vi "Flush Control Value.vi"(4 "error in (no error)":errorcluster, 5 "Tab Control Ref In":T2, 6 "Tree Control In":refnum<vi>, 7 "Session In":T1) -> (0 "error out":errorcluster, 2 "Tree Control Out":refnum<vi>, 3 "Session Out":T1)   [LabVIEW 2012]
doc: "The Flush Control Value subVI reads the value of the control, and then sets the value of the attribute in the IMAQdx driver."
uses:
  <vilib>/userDefined/High Color/IMAQdx.ctl
  <vilib>/vision/driver/IMAQdx.llb/IMAQdx Attribute Type.ctl
  <vilib>/vision/driver/NI_Vision_Acquisition_Software.lvlib
  <resource>/objmgr/imaqdx.rc
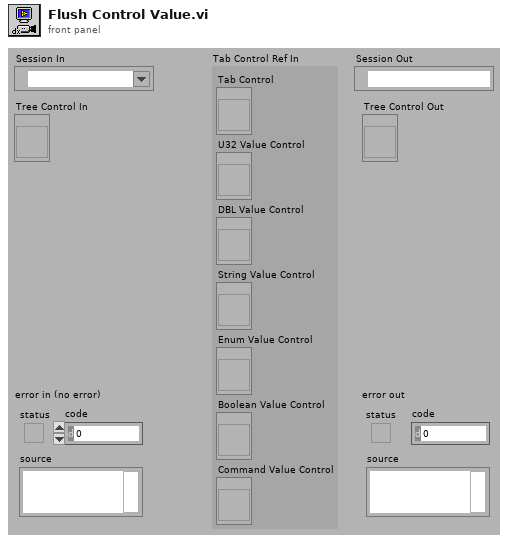
[diagram p1: front panel]
types:
  T1 = typedef "IMAQdx.ctl" = refnum<k21>
  T2 = cluster{"Tab Control":refnum<vi>, "U32 Value Control":refnum<vi>, "DBL Value Control":refnum<vi>, "String Value Control":refnum<vi>, "Enum Value Control":refnum<vi>, "Boolean Value Control":refnum<vi>, "Command Value Control":refnum<vi>}
  T3 = typedef "NI_Vision_Acquisition_Software.lvlib/IMAQdx Attribute Type.ctl" = enum32{"U32", "I64", "DBL", "String", "Enum", "Bool", "Command"}
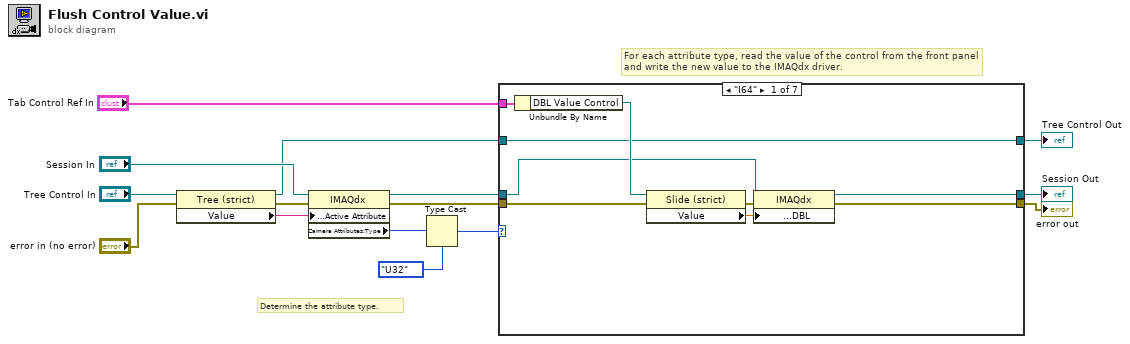
[diagram p0: block diagram]
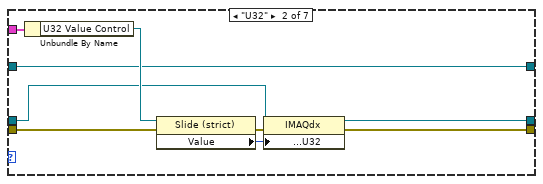
[diagram p2: hidden frame]
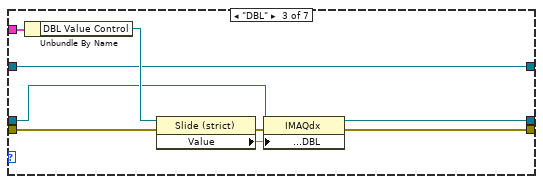
[diagram p3: hidden frame]
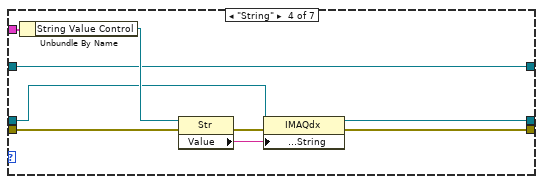
[diagram p4: hidden frame]
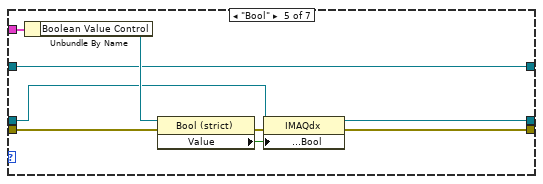
[diagram p5: hidden frame]
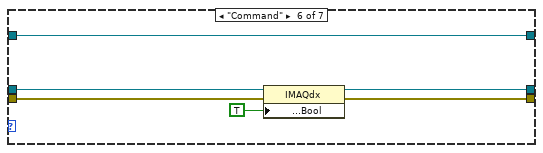
[diagram p6: hidden frame]
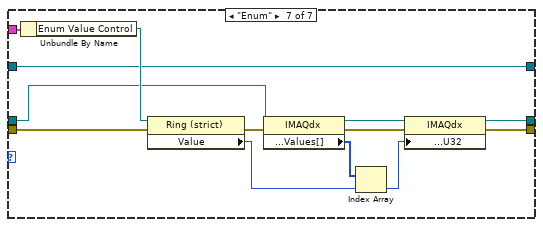
[diagram p7: hidden frame]
diagram:
  # "For each attribute type, read the value of the control from the front panel\nand write the new value to the IMAQdx driver."
  # "Determine the attribute type."
  n1 = property class="Tree (strict)"(reference="Tree Control In", error in="error in (no error)") -> (reference out=w4:refnum<vi>, error out=w13:errorcluster, "Value"=w11:string)
  n2 = property class="IMAQdx"(reference="Session In", error in=w13, "Camera Attributes:Active Attribute"=w11) -> (reference out=w6:T1, error out=w7:errorcluster, "Camera Attributes:Type"=w10:u32)
  n3 = Type Cast(type=IMAQdx_Attribute_Type."U32" ("Attribute Type"), x=w10) -> (*(type *) &x=w8:T3)
  n4 = case shown="\"I64\"" w8 {
    tunnel: w7 -> [w22 w31 w40 w49 w58 w62 w77]
    tunnel: w6 -> [w20 w29 w38 w47 w56 w66 w75]
    tunnel: "Tab Control Ref In" -> [w24 w33 w42 w51 w60 _ w79]
    tunnel: [w18 w27 w36 w45 w54 w65 w73] -> w2
    tunnel: [w17 w26 w35 w44 w53 w64 w72] -> w1
    tunnel: [w16 w25 w34 w43 w52 w63 w74] -> w3
    tunnel: w4 -> [w16 w25 w34 w43 w52 w63 w74]
    frame "I64" {
      n5 = Unbundle By Name(w24) -> ("DBL Value Control"=w23:refnum<vi>)
      n6 = property class="Slide (strict)"(reference=w23, error in=w22) -> (error out=w21:errorcluster, "Value"=w19:dbl)  [unwired: 1 out]
      n7 = property class="IMAQdx"(reference=w20, error in=w21, "Camera Attributes:Value:DBL"=w19) -> (reference out=w18:T1, error out=w17:errorcluster)
    }
    frame "U32" {
      n8 = Unbundle By Name(w33) -> ("U32 Value Control"=w32:refnum<vi>)
      n9 = property class="Slide (strict)"(reference=w32, error in=w31) -> (error out=w30:errorcluster, "Value"=w28:u32)  [unwired: 1 out]
      n10 = property class="IMAQdx"(reference=w29, error in=w30, "Camera Attributes:Value:U32"=w28) -> (reference out=w27:T1, error out=w26:errorcluster)
    }
    frame "DBL" {
      n11 = Unbundle By Name(w42) -> ("DBL Value Control"=w41:refnum<vi>)
      n12 = property class="Slide (strict)"(reference=w41, error in=w40) -> (error out=w39:errorcluster, "Value"=w37:dbl)  [unwired: 1 out]
      n13 = property class="IMAQdx"(reference=w38, error in=w39, "Camera Attributes:Value:DBL"=w37) -> (reference out=w36:T1, error out=w35:errorcluster)
    }
    frame "String" {
      n14 = Unbundle By Name(w51) -> ("String Value Control"=w50:refnum<vi>)
      n15 = property class="Str"(reference=w50, error in=w49) -> (error out=w48:errorcluster, "Value"=w46:string)  [unwired: 1 out]
      n16 = property class="IMAQdx"(reference=w47, error in=w48, "Camera Attributes:Value:String"=w46) -> (reference out=w45:T1, error out=w44:errorcluster)
    }
    frame "Bool" {
      n17 = Unbundle By Name(w60) -> ("Boolean Value Control"=w59:refnum<vi>)
      n18 = property class="Bool (strict)"(reference=w59, error in=w58) -> (error out=w57:errorcluster, "Value"=w55:bool)  [unwired: 1 out]
      n19 = property class="IMAQdx"(reference=w56, error in=w57, "Camera Attributes:Value:Bool"=w55) -> (reference out=w54:T1, error out=w53:errorcluster)
    }
    frame "Command" {
      n20 = property class="IMAQdx"(reference=w66, error in=w62, "Camera Attributes:Value:Bool"=TRUE ("ValueBool")) -> (reference out=w65:T1, error out=w64:errorcluster)
    }
    frame "Enum" {
      n21 = Unbundle By Name(w79) -> ("Enum Value Control"=w78:refnum<vi>)
      n22 = property class="Ring (strict)"(reference=w78, error in=w77) -> (error out=w76:errorcluster, "Value"=w67:u32)  [unwired: 1 out]
      n23 = property class="IMAQdx"(reference=w75, error in=w76) -> (reference out=w71:T1, error out=w70:errorcluster, "Camera Attributes:Enum:Values[]"=w69:u32[])
      n24 = Index Array(array=w69, index=w67) -> (element=w68:u32)
      n25 = property class="IMAQdx"(reference=w71, error in=w70, "Camera Attributes:Value:U32"=w68) -> (reference out=w73:T1, error out=w72:errorcluster)
    }
  }
  "Tree Control Out" <- w3
  "Session Out" <- w2
  "error out" <- w1
